vi "JSON to Cluster.vi"(8 "error in":errorcluster, 11 "JSON String":string="{\n    \"firstName\": \"John\",\n    \"lastName\": \"Smith\",\n    \"age\": 25,\n    \"address\": {\n        \"streetAddress\": \"21 2nd Street\",\n        \"city\": \"New York\",\n        \"state\": \"NY\",\n        \"postalCode\": 10021\n    },\n    \"phoneNumbers\": [\n        {\n            \"type\": \"home\",\n            \"number\": \"212 555-1234\"\n        },\n        {\n            \"type\": \"fax\",\n            \"number\": \"646 555-4567\"\n        }\n    ]\n}") -> (0 "error out":errorcluster)   [LabVIEW 2013]
uses:
  <vilib>/ErrorRing/Error Ring.xnode
  <vilib>/Utility/error.llb/Error Cluster From Error Code.vi
panel:
  # "1. Paste JSON string into control and run VI\n2. New VI is created that contains cluster \nrepresentation of the object, and that can\nbe used with the Unflatten from JSON VI"
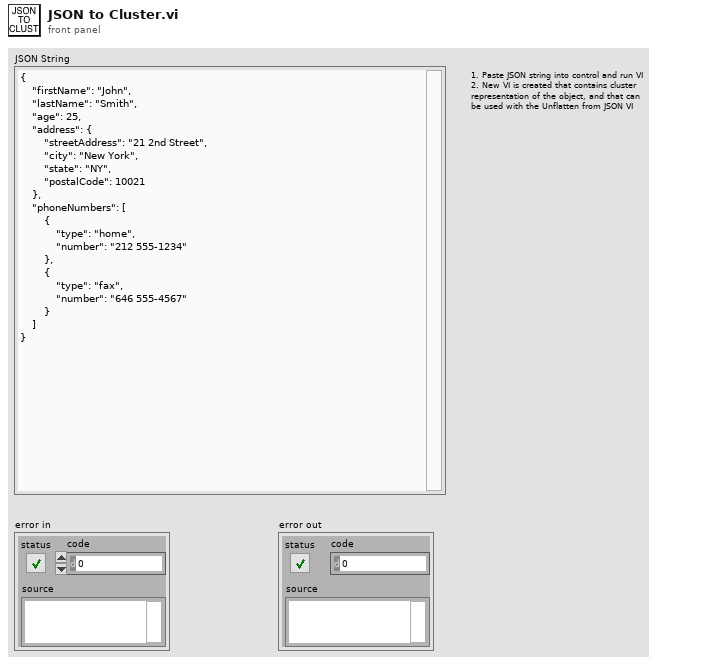
[diagram p1: front panel]
types:
  T1 = typedef "Token.ctl" = enum16{"End", "Boolean", "Named Cluster", "Unnamed Cluster", "Array", "String", "Decimal", "FloatingPoint", "End Array", "End Cluster"}
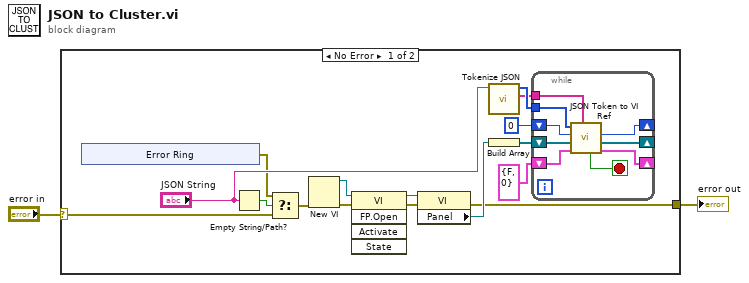
[diagram p0: block diagram]
diagram:
  n1 = case shown="No Error" "error in" {
    selector: "error in" -> [w6 w33]
    tunnel: [w3 w33] -> w1
    frame No Error {
      n2 = xnode "Error Ring"() -> ("error out"=w5:errorcluster)
      n3 = Empty String/Path?(string/path="JSON String") -> (empty?=w8:bool)
      n4 = Select(t=w5, s=w8, f=w6) -> (s? t:f=w4:errorcluster)
      n5 = New VI(8:w4) -> (0:w10:errorcluster, 3:w9:refnum<vi>)  [unwired: 6 in]
      n6 = invoke class="VI" method="FP.Open"(reference=w9, error in=w10) -> (reference out=w15:refnum<vi>, error out=w13:errorcluster)  [unwired: 3 in, 3 out]
      n7 = property class="VI"(reference=w15, error in=w13) -> (error out=w3:errorcluster, "Panel"=w14:refnum<vi>)  [unwired: 1 out]
      n8 = call "Tokenize JSON.vi"("JSON String"="JSON String") -> ("Variable Names"=w17:string[], "Token Array"=w18:T1[])  [unwired: 9 in]
      n9 = Build Array(w14) -> (w11:refnum<vi>[])
      n10 = while {
        tunnel: w18 -> [w31]
        tunnel: w17 -> [w30]
        shift-right: [w28] -> _
        shift-left: 0 -> [w29]
        shift-right: [w27] -> _
        shift-left: w11 -> [w32]
        shift-right: [w24] -> _
        shift-left: cluster{"In Array?":bool, "Cluster Level":i32} {"In Array?"=FALSE, "Cluster Level"=0} ("Inception Tracking") -> [w25]
        stop <- w26 stop-if-true
        n11 = call "JSON Token to VI Ref.vi"("Variable Names"=w30, "Inception Tracking"=w25, "Parent Ref"=w32, "index"=w29, "Token Array"=w31) -> ("Inception Tracking Out"=w24:cluster{"In Array?":bool, "Cluster Level":i32}, "Parent Ref Out"=w27:refnum<vi>[], "index out"=w28:i32, "End?"=w26:bool)  [unwired: 3 in]
      }
    }
    frame Error {
    }
  }
  "error out" <- w1
